vi "Instrument.OxfordVRM.FloatApprox (Array).vi"(4 "y":dbl[](array[numeric]), 5 "x":dbl[](array[numeric])) -> (1 "x ~ y?":bool)   [LabVIEW 2019, in "Instrument.OxfordVRM.lvclass"]
doc: "Use to compare floating point numbers. This will check if two numbers are the same to 6 decimal places. Edit block diagram to change tolerance."
uses:
  Instrument.OxfordVRM.lvclass
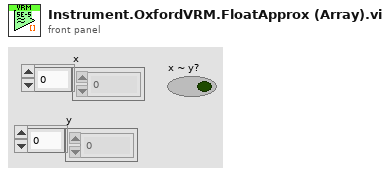
[diagram p1: front panel]
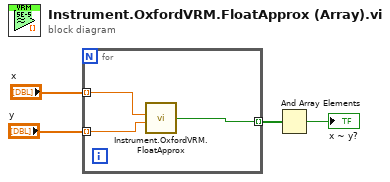
[diagram p0: block diagram]
diagram:
  n1 = for {
    tunnel: [w5] -> w4 mode=indexing
    tunnel: "y" -> [w6] mode=indexing
    tunnel: "x" -> [w7] mode=indexing
    n2 = call "Instrument.OxfordVRM.FloatApprox.vi"("y"=w6, "x"=w7) -> ("x ~ y?"=w5:bool)  [unwired: 4 in]
  }
  n3 = And Array Elements(Boolean array=w4) -> (logical AND=→"x ~ y?":bool)
